vi "NMIdleLoop.vi"(0 "mx task in":refnum<k21>, 1 "ULx task in":refnum<k24>, 2 "Tab Control":enum32{"ULx", "DAQmx"}(tab), 5 "error in":errorcluster, 6 "Start":bool, 8 "ExStop":bool, 10 "ExClear":bool) -> (7 "Task Start":bool, 9 "Task Stop":bool, 11 "Task Clear":bool, 14 "mx task out":refnum<k21>, 15 "ULx task out":refnum<k24>, 16 "Name":refnum<k21>, 17 "Task":i32 format="%x", 18 "Function":i32, 19 "error out":errorcluster)   [LabVIEW 2010]
uses:
  C:/Program Files/National Instruments/LabVIEW 2010/vi.lib/ULx/ULx_LV.dll
  Program Files/National Instruments/LabVIEW 2010/vi.lib/ULx/ULx_LV.dll
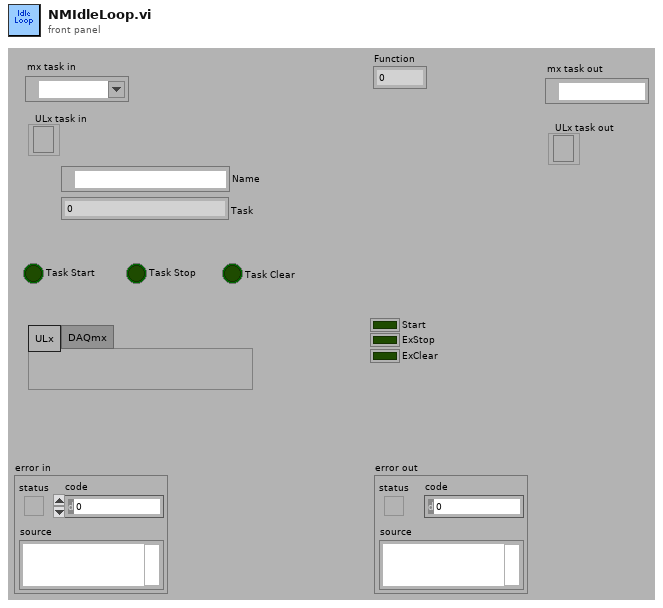
[diagram p1: front panel]
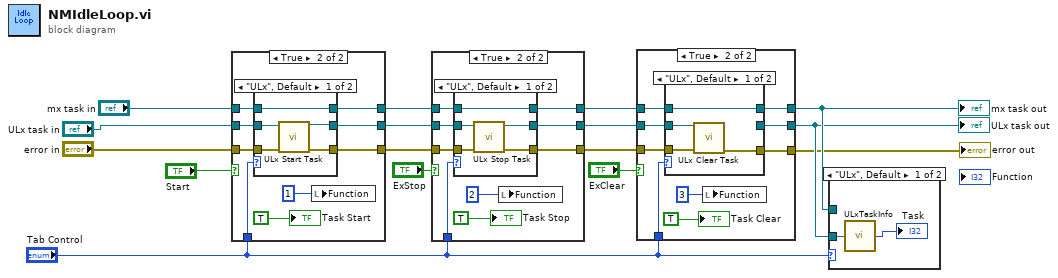
[diagram p0: block diagram]
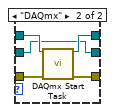
[diagram p3: hidden frame]
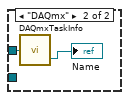
[diagram p4: hidden frame]
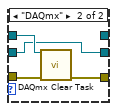
[diagram p6: hidden frame]
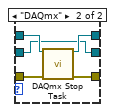
[diagram p8: hidden frame]
diagram:
  n1 = case shown="True" "Start" {
    tunnel: [w19 w28] -> w2
    tunnel: "ULx task in" -> [w19 w27]
    tunnel: "error in" -> [w18 w26]
    tunnel: [w18 w25] -> w3
    tunnel: "mx task in" -> [w17 w23]
    tunnel: "Tab Control" -> [_ w24]
    tunnel: [w17 w22] -> w1
    frame False {
    }
    frame True {
      n2 = case shown="\"ULx\", Default" w24 {
        tunnel: [w33 w34] -> w28
        tunnel: w27 -> [w32 w34]
        tunnel: w26 -> [w31 w37]
        tunnel: [w30 w38] -> w25
        tunnel: w23 -> [w29 w36]
        tunnel: [w29 w35] -> w22
        frame "ULx", Default {
          n3 = call <vilib>:"ULx Start Task.vi"("task in"=w32, "error in"=w31) -> ("task out"=w33:refnum<k24>, "error out"=w30:errorcluster)  [unwired: 12 in]
        }
        frame "DAQmx" {
          n4 = call <vilib>:"DAQmx Start Task.vi"("task/channels in"=w36, "error in"=w37) -> ("task out"=w35:refnum<k21>, "error out"=w38:errorcluster)  [unwired: 12 in]
        }
      }
      n5 = local write "Function"(1) -> ()
      "Task Start" <- TRUE
    }
  }
  n6 = case shown="True" "ExStop" {
    tunnel: [w41 w50] -> w8
    tunnel: w2 -> [w41 w49]
    tunnel: w3 -> [w40 w48]
    tunnel: [w40 w47] -> w7
    tunnel: w1 -> [w39 w45]
    tunnel: "Tab Control" -> [_ w46]
    tunnel: [w39 w44] -> w9
    frame False {
    }
    frame True {
      n7 = case shown="\"ULx\", Default" w46 {
        tunnel: [w55 w56] -> w50
        tunnel: w49 -> [w54 w56]
        tunnel: w48 -> [w53 w59]
        tunnel: [w52 w60] -> w47
        tunnel: w45 -> [w51 w58]
        tunnel: [w51 w57] -> w44
        frame "ULx", Default {
          n8 = call <vilib>:"ULx Stop Task.vi"("error in"=w53, "task in"=w54) -> ("error out"=w52:errorcluster, "task out"=w55:refnum<k24>)  [unwired: 8 in]
        }
        frame "DAQmx" {
          n9 = call <vilib>:"DAQmx Stop Task.vi"("task/channels in"=w58, "error in"=w59) -> ("task out"=w57:refnum<k21>, "error out"=w60:errorcluster)  [unwired: 12 in]
        }
      }
      n10 = local write "Function"(2) -> ()
      "Task Stop" <- TRUE
    }
  }
  n11 = case shown="True" "ExClear" {
    tunnel: w8 -> [w61 w72]
    tunnel: w7 -> [w63 w71]
    tunnel: [w63 w70] -> w5
    tunnel: "Tab Control" -> [_ w69]
    tunnel: w9 -> [w62 w68]
    tunnel: [w62 w67] -> w12
    tunnel: [w61 w66] -> w11
    frame False {
    }
    frame True {
      n12 = case shown="\"ULx\", Default" w69 {
        tunnel: w72 -> [w76 w77]
        tunnel: w71 -> [w75 w79]
        tunnel: [w74 w80] -> w70
        tunnel: w68 -> [w73 w78]
        tunnel: [w73 _] -> w67
        tunnel: [_ w77] -> w66
        frame "ULx", Default {
          n13 = call <vilib>:"ULx Clear Task.vi"("task in"=w76, "error in"=w75) -> ("error out"=w74:errorcluster)  [unwired: 13 in]
        }
        frame "DAQmx" {
          n14 = call <vilib>:"DAQmx Clear Task.vi"("task in"=w78, "error in"=w79) -> ("error out"=w80:errorcluster)  [unwired: 13 in]
        }
      }
      n15 = local write "Function"(3) -> ()
      "Task Clear" <- TRUE
    }
  }
  "mx task out" <- w12
  "ULx task out" <- w11
  "error out" <- w5
  n16 = case shown="\"ULx\", Default" "Tab Control" {
    tunnel: w11 -> [w82 _]
    tunnel: w12 -> [_ w84]
    frame "ULx", Default {
      n17 = call "ULxTaskInfo.vi"("task in"=w82) -> ("Task"=→"Task":i32)  [unwired: 2 out]
    }
    frame "DAQmx" {
      n18 = call "DAQmxTaskInfo.vi"("task in"=w84) -> ("Name"=→"Name":refnum<k21>)  [unwired: 1 out]
    }
  }
